vi "Aim With Vision.vi"(2 "Aim":bool, 3 "Gyro Angle":dbl=-0.0007054623688) -> (0 "Ready":bool, 1 "Checked Image":bool)   [LabVIEW 2012]
uses:
  Robot Global Data.vi
  <vilib>/Rock Robotics/WPI/Joystick/WPI_JoystickGetSetRefNum.vi
panel:
  in  "Aim Position":dbl=60.0
  out "Shooter Speed":dbl=10.0
  out "High Target Index":i32
  in  "Open Position":dbl=90.0
  in  "Closed Position":dbl
  in  "Rest Speed r/s":dbl=15.0 min=0.0 max=0.7 step=0.05
  in  "Aiming Tolerance (Deg)":dbl=2.0
  # "25"
  # "2"
  # "0"
  # "Gate Servo"
  # "60"
  # "90"
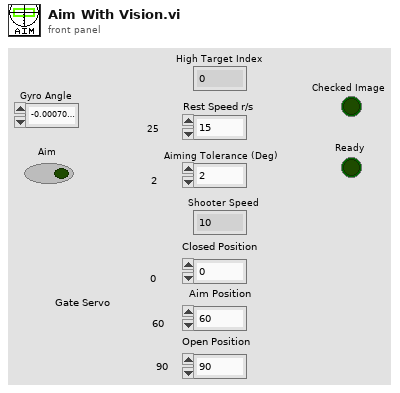
[diagram p1: front panel]
types:
  T1 = typedef "WPI_JoystickDevRef.ctl" = cluster{"Device":T2}
  T2 = typedef "WPI_JoystickDeviceEnum.ctl" = enum16{"USB 1", "USB 2", "USB 3", "USB 4", "Kinect 1", "Kinect 2"}
  T3 = typedef "WPI_JoystickButtonState.ctl" = cluster{"Button 1":bool, "Button 2":bool, "Button 3":bool, "Button 4":bool, "Button 5":bool, "Button 6":bool, "Button 7":bool, "Button 8":bool, "Button 9":bool, "Button 10":bool, "Button 11":bool, "Button 12":bool}
  T4 = cluster{"Center Position":cluster{"X":dbl, "Y":dbl}, "Distance (ft)":dbl, "Center":bool}[]
  T5 = typedef "WPI_ServoDeviceRef.ctl" = cluster{"DeviceStatus":errorcluster, "Digital Module":T6, "PWM Channel":T7, "DeadBand":T8}
  T6 = typedef "FPGA_TypedefDigitalModule.ctl" = enum16{"Digital Module 1", "Digital Module 2"}
  T7 = typedef "FPGA_DIOPWMChannel.ctl" = enum8{"PWM 1", "PWM 2", "PWM 3", "PWM 4", "PWM 5", "PWM 6", "PWM 7", "PWM 8", "PWM 9", "PWM 10", "Invalid"}
  T8 = typedef "WPI_PWMDeadband.ctl" = cluster{"Name":string, "maxPositivePwm":i32, "minPositivePwm":i32, "centerPwm":i32, "maxNegativePwm":i32, "minNegativePwm":i32, "angularRange":u16}
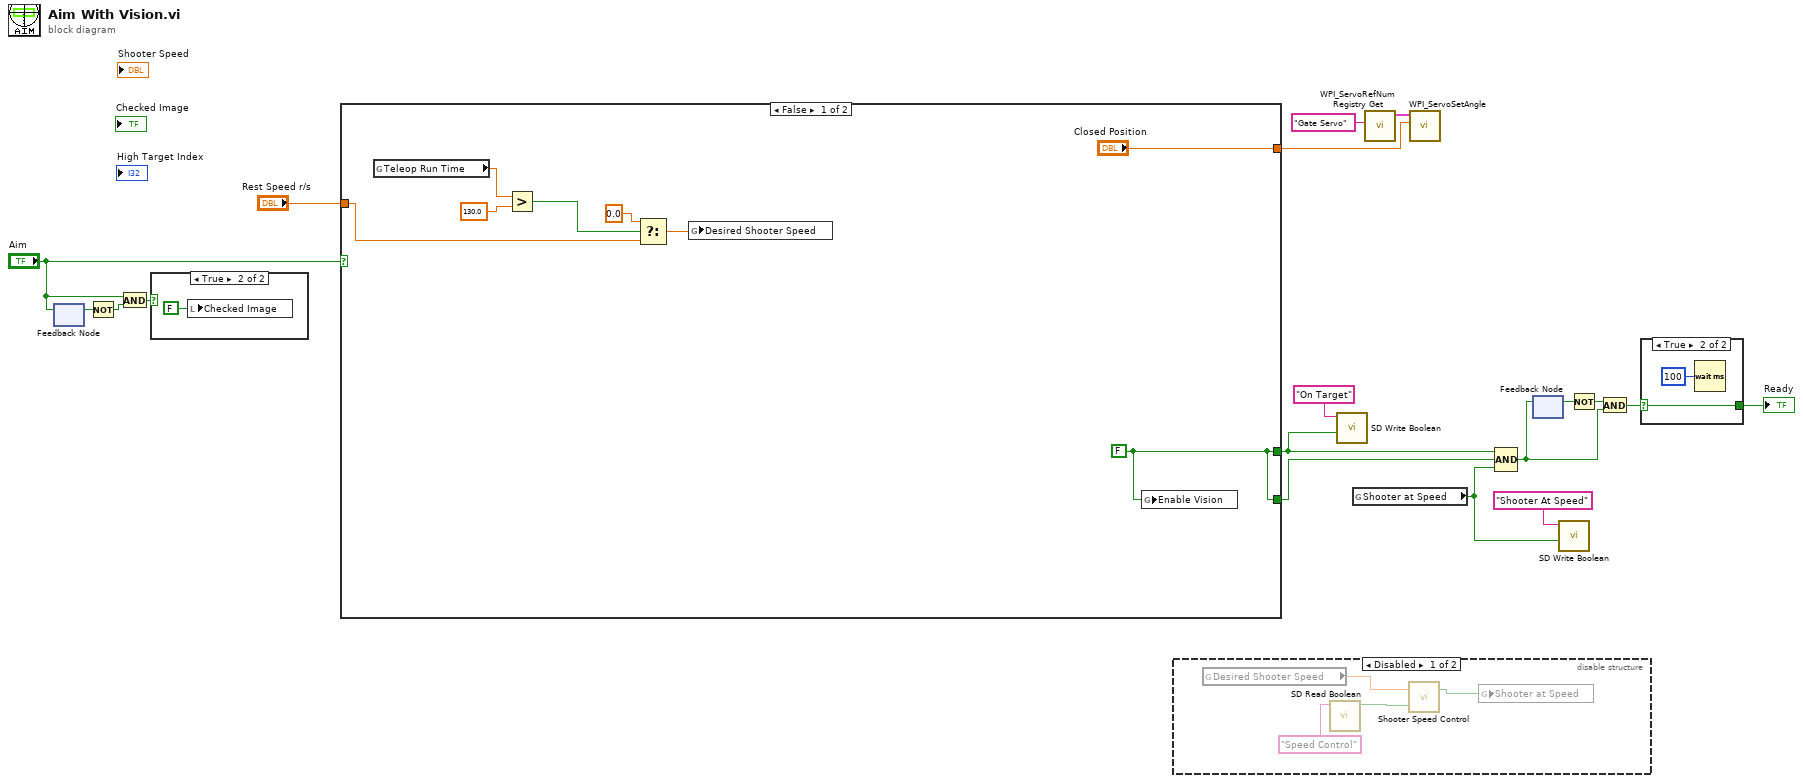
[diagram p0: block diagram]
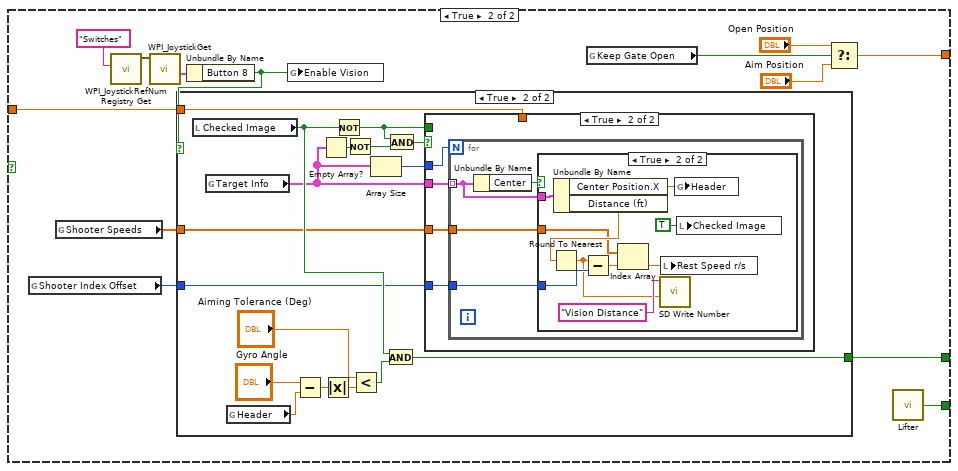
[diagram p5: hidden frame]
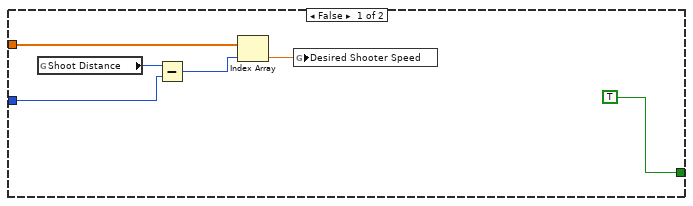
[diagram p6: hidden frame]
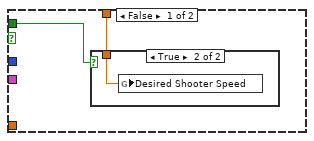
[diagram p7: hidden frame]
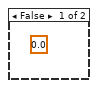
[diagram p9: hidden frame]
diagram:
  n1 = feedback-in #1("Aim") -> ()
  n2 = feedback #1() -> (w11:bool)  [unwired: 1 in]
  n3 = Not(x=w11) -> (.not. x?=w9:bool)
  n4 = And(x="Aim", y=w9) -> (x .and. y?=w12:bool)
  n5 = case shown="True" w12 {
    frame False {
    }
    frame True {
      n6 = local write "Checked Image"(FALSE ("Checked Image")) -> ()
    }
  }
  n7 = case shown="False" "Aim" {
    tunnel: [w26 w40] -> w7
    tunnel: ["Closed Position" w34] -> w16
    tunnel: "Rest Speed r/s" -> [w21 w39]
    tunnel: [w26 w30] -> w8
    frame False {
      w26 = FALSE
      n8 = global read "Robot Global Data.vi" "Teleop Run Time"() -> (w25:dbl)
      n9 = Greater?(x=w25, y=130.0) -> (0:w23:bool)
      n10 = Select(t=0.0, s=w23, f=w21) -> (s? t:f=w20:dbl)
      n11 = global write "Robot Global Data.vi" "Desired Shooter Speed"(w20) -> ()
      n12 = global write "Robot Global Data.vi" "Enable Vision"(w26) -> ()
    }
    frame True {
      n13 = global read "Robot Global Data.vi" "Shooter Index Offset"() -> (w28:i32)
      n14 = global read "Robot Global Data.vi" "Shooter Speeds"() -> (w29:dbl[])
      n15 = call <vilib>:"WPI_JoystickRefNum Registry Get.vi"("refnum name"="Switches") -> ("JoystickDevRef"=w37:T1)  [unwired: 1 in, 9 out]
      n16 = call <vilib>:"WPI_JoystickGet.vi"("JoystickDevRef"=w37) -> ("Buttons"=w36:T3)  [unwired: 1 in, 5 out]
      n17 = Unbundle By Name(w36) -> ("Button 8"=w35:bool)
      n18 = case shown="True" w35 {
        tunnel: [TRUE w55] -> w40
        tunnel: w29 -> [w45 w49]
        tunnel: w28 -> [w43 w50]
        tunnel: w39 -> [_ w47]
        frame False {
          n19 = global read "Robot Global Data.vi" "Shoot Distance"() -> (w42:i32)
          n20 = Subtract(x=w42, y=w43) -> (x-y=w44:i32)
          n21 = Index Array(array=w45, index=w44) -> (element=w41:dbl)
          n22 = global write "Robot Global Data.vi" "Desired Shooter Speed"(w41) -> ()
        }
        frame True {
          n23 = local read "Checked Image"() -> (w59:bool)
          n24 = global read "Robot Global Data.vi" "Target Info"() -> (w53:T4)
          n25 = global read "Robot Global Data.vi" "Header"() -> (w61:dbl)
          n26 = Subtract(x="Gyro Angle", y=w61) -> (x-y=w58:dbl)
          n27 = Empty Array?(array=w53) -> (empty?=w63:bool)
          n28 = Absolute Value(x=w58) -> (abs(x)=w54:dbl)
          n29 = Not(x=w59) -> (.not. x?=w48:bool)
          n30 = Not(x=w63) -> (.not. x?=w51:bool)
          n31 = Less?(x="Aiming Tolerance (Deg)", y=w54) -> (x < y?=w56:bool)
          n32 = Array Size(array=w53) -> (size(s)=w52:i32)
          n33 = And(x=w59, y=w56) -> (x .and. y?=w55:bool)
          n34 = And(x=w48, y=w51) -> (x .and. y?=w62:bool)
          n35 = case shown="True" w62 {
            tunnel: w53 -> [_ w69]
            tunnel: w52 -> [_ w70]
            tunnel: w50 -> [_ w68]
            tunnel: w49 -> [_ w67]
            tunnel: w48 -> [w65 _]
            tunnel: w47 -> [w64 _]
            frame False {
              n36 = case shown="True" w65 {
                tunnel: w64 -> [_ w66]
                frame False {
                }
                frame True {
                  n37 = global write "Robot Global Data.vi" "Desired Shooter Speed"(w66) -> ()
                }
              }
            }
            frame True {
              n38 = for {
                N: w70 -> [_]
                tunnel: w69 -> [w73] mode=indexing
                tunnel: w68 -> [w72]
                tunnel: w67 -> [w71]
                n39 = Unbundle By Name(w73) -> ("Center"=w74:bool)
                n40 = case shown="True" w74 {
                  tunnel: w73 -> [_ w83]
                  tunnel: w72 -> [_ w81]
                  tunnel: w71 -> [_ w79]
                  frame False {
                    (unwired) 0.0 ("Numeric")
                  }
                  frame True {
                    n41 = Unbundle By Name(w83) -> ("Center Position.X"=w84:dbl, "Distance (ft)"=w82:dbl)
                    n42 = Round To Nearest(number=w82) -> (nearest integer value=w75:dbl)
                    n43 = Subtract(x=w75, y=w81) -> (x-y=w80:dbl)
                    n44 = Index Array(array=w79, index=w80) -> (element=w78:dbl)
                    n45 = call <vilib>:"SD Write Number.vi"("Numeric"=w75, "Name"="Vision Distance") -> ()  [unwired: 8 in, 2 out]
                    n46 = local write "Rest Speed r/s"(w78) -> ()
                    n47 = global write "Robot Global Data.vi" "Header"(w84) -> ()
                    n48 = local write "Checked Image"(TRUE ("Read Angle")) -> ()
                  }
                }
              }
            }
          }
        }
      }
      n49 = global write "Robot Global Data.vi" "Enable Vision"(w35) -> ()
      n50 = global read "Robot Global Data.vi" "Keep Gate Open"() -> (w31:bool)
      n51 = Select(t="Open Position", s=w31, f="Aim Position") -> (s? t:f=w34:dbl)
      n52 = call "Lifter.vi"() -> ("In Position"=w30:bool)  [unwired: 1 in]
    }
  }
  n53 = disable-structure shown="Disabled" {
    frame Disabled {
      n54 = global read "Robot Global Data.vi" "Desired Shooter Speed"() -> (w85:dbl)
      n55 = call <vilib>:"SD Read Boolean.vi"("Name"="Speed Control") -> ("Boolean"=w87:bool)  [unwired: 8 in, 2 out]
      n56 = call "Shooter Speed Control.vi"("Use Speed Control"=w87, "Desired\nShooter\nSpeed"=w85) -> ("up to speed"=w86:bool)  [unwired: 1 in]
      n57 = global write "Robot Global Data.vi" "Shooter at Speed"(w86) -> ()
    }
    frame Enabled {
    }
  }
  n58 = call <vilib>:"SD Write Boolean.vi"("Boolean"=w7, "Name"="On Target") -> ()  [unwired: 8 in, 2 out]
  n59 = global read "Robot Global Data.vi" "Shooter at Speed"() -> (w2:bool)
  n60 = call <vilib>:"WPI_ServoRefNum Registry Get.vi"("refnum name"="Gate Servo") -> ("ServoDeviceRef"=w18:T5)  [unwired: 9 in, 1 out]
  n61 = call <vilib>:"WPI_ServoSetAngle.vi"("Angle"=w16, "ServoDeviceRef"=w18) -> ()  [unwired: 8 in, 2 out]
  n62 = Compound Arithmetic op=AND(w7, w8, w2) -> (w3:bool)
  n63 = feedback-in #2(w3) -> ()
  n64 = feedback #2() -> (w5:bool)  [unwired: 1 in]
  n65 = call <vilib>:"SD Write Boolean.vi"("Boolean"=w2, "Name"="Shooter At Speed") -> ()  [unwired: 8 in, 2 out]
  n66 = Not(x=w5) -> (.not. x?=w4:bool)
  n67 = And(x=w4, y=w3) -> (x .and. y?=w6:bool)
  n68 = case shown="True" w6 {
    selector: w6 -> [w89 w90]
    tunnel: [w89 w90] -> w1
    frame False {
    }
    frame True {
      n69 = Wait (ms)(milliseconds to wait=u32 100) -> ()  [unwired: 1 out]
    }
  }
  "Ready" <- w1
